vi "CFTS-Build All.vi"() -> ()   [LabVIEW 2020]
uses:
  <vilib>/AppBuilder/AB_API_Simple/Build (path).vi
  <vilib>/AppBuilder/AB_API_Simple/NI_App_Builder_API.lvlib
panel:
  in  "stop":bool
  out "Progress Bar":u8(slide) caption="Error" scale=0.0..2.0
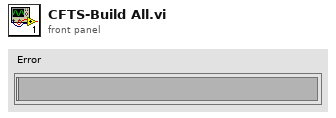
[diagram p1: front panel]
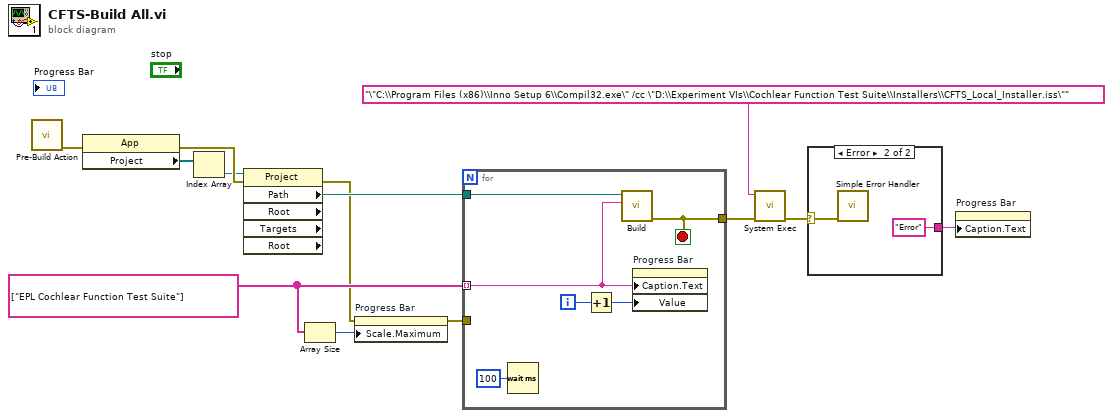
[diagram p0: block diagram]
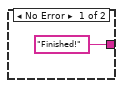
[diagram p2: hidden frame]
diagram:
  w2 = string[] ["EPL Cochlear Function Test Suite"]
  n1 = call "Pre-Build Action.vi"() -> ("error out"=w9:errorcluster)  [unwired: 11 in]
  n2 = property class="App"(error in=w9) -> (error out=w13:errorcluster, "Project"=w12:refnum<vi>[])  [unwired: 1 in, 1 out]
  n3 = Index Array(array=w12) -> (element=w11:refnum<vi>)  [unwired: 1 in]
  n4 = property class="Project" props=["Path", "Root", "Targets", "Root"](reference=w11, error in=w13) -> (error out=w1:errorcluster, "Path"=w10:path)  [unwired: 4 out]
  n5 = Array Size(array=w2) -> (size(s)=w8:i32)
  n6 = property on="Progress Bar" class="Slide (strict)"(error in=w1, "Scale.Maximum"=w8) -> (error out=w7:errorcluster)  [unwired: 1 in, 1 out]
  n7 = for {
    tunnel: w10 -> [w19]
    tunnel: w2 -> [w14] mode=indexing
    tunnel: [w15] -> w4
    tunnel: w7 -> [_]
    i -> [w18]
    stop <- w15 stop-if-true
    n8 = Wait (ms)(milliseconds to wait=u32 100) -> ()  [unwired: 1 out]
    n9 = Increment(x=w18) -> (x+1=w17:i32)
    n10 = call-poly <vilib>:"Build.vi"("Name of build specification (if empty: build all)"=w14, "Path to project"=w19) -> ("error out"=w15:errorcluster)  [unwired: 8 in, 1 out]
    n11 = property on="Progress Bar" class="Slide (strict)"("Caption.Text"=w14, "Value"=w17) -> ()  [unwired: 2 in, 2 out]
  }
  n12 = call <vilib>:"System Exec.vi"("error in (no error)"=w4, "command line"="\"C:\\Program Files (x86)\\Inno Setup 6\\Compil32.exe\" /cc \"D:\\Experiment VIs\\Cochlear Function Test Suite\\Installers\\CFTS_Local_Installer.iss\"") -> ("error out"=w3:errorcluster)  [unwired: 6 in, 3 out]
  n13 = case shown="Error" w3 {
    selector: w3 -> [_ w21]
    tunnel: ["Finished!" "Error"] -> w6
    frame No Error {
    }
    frame Error {
      n14 = call <vilib>:"Simple Error Handler.vi"("error in (no error)"=w21) -> ()  [unwired: 4 in, 5 out]
    }
  }
  n15 = property on="Progress Bar" class="Slide (strict)"("Caption.Text"=w6) -> ()  [unwired: 2 in, 2 out]
